vi "Get Multi.vi"(0 "Display State In":T2, 5 "Value In":T1, 9 "Container State":T3, 11 "error in (no error)":errorcluster) -> (4 "Display State Out":T2, 6 "Value Out":T1, 15 "error out":errorcluster)   [LabVIEW 2015, in "Tone (G3).xctl"]
uses:
  Tone (G3).xctl
  <vilib>/_xctls/Container State.ctl
  State.ctl
  Utility VIs/Controls/KNumeric (DBL)/KNumeric (DBL).xctl
  Utility VIs/Controls/KCheckbox/KCheckbox.xctl
  Tone.Properties.ctl
  <vilib>/_xctls/XControlSupport.lvlib
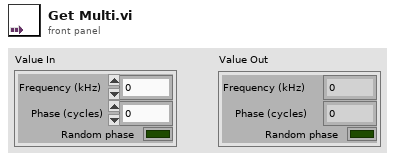
[diagram p1: front panel]
types:
  T1 = typedef "Tone (G3).xctl/Tone.Properties.ctl" = cluster{"Frequency (kHz)":dbl, "Phase (cycles)":dbl, "Random phase":bool}
  T2 = typedef "Tone (G3).xctl/State.ctl" = cluster{"enable menu":bool, "ctls":cluster{"Freq":refnum<vi>, "Phase":refnum<vi>, "Random":refnum<vi>}}
  T3 = typedef "XControlSupport.lvlib/Container State.ctl" = cluster{"Indicator?":bool, "Run Mode?":bool, " Refnum":refnum<vi>}
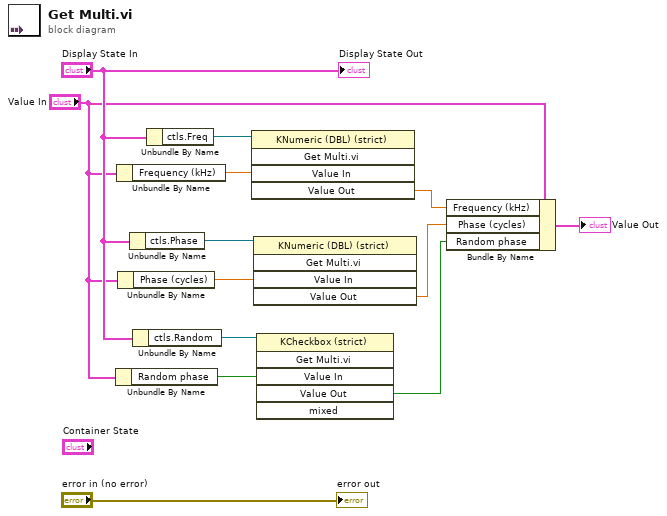
[diagram p0: block diagram]
diagram:
  n1 = Unbundle By Name("Value In") -> ("Random phase"=w2:bool)
  n2 = Unbundle By Name("Value In") -> ("Frequency (kHz)"=w9:dbl)
  n3 = Unbundle By Name("Value In") -> ("Phase (cycles)"=w7:dbl)
  n4 = Unbundle By Name("Display State In") -> ("ctls.Phase"=w11:refnum<vi>)
  n5 = Unbundle By Name("Display State In") -> ("ctls.Random"=w3:refnum<vi>)
  n6 = Unbundle By Name("Display State In") -> ("ctls.Freq"=w10:refnum<vi>)
  n7 = invoke class="KNumeric (DBL) (strict)" method="Get Multi.vi"(reference=w10, "Value In"=w9) -> ("Value Out"=w8:dbl)  [unwired: 3 in, 4 out]
  n8 = invoke class="KNumeric (DBL) (strict)" method="Get Multi.vi"(reference=w11, "Value In"=w7) -> ("Value Out"=w6:dbl)  [unwired: 3 in, 4 out]
  n9 = invoke class="KCheckbox (strict)" method="Get Multi.vi"(reference=w3, "Value In"=w2) -> ("Value Out"=w1:bool)  [unwired: 4 in, 5 out]
  n10 = Bundle By Name(cluster="Value In", "Frequency (kHz)"=w8, "Phase (cycles)"=w6, "Random phase"=w1) -> (→"Value Out":T1)
  "Display State Out" <- "Display State In"
  "error out" <- "error in (no error)"
